vi "ToDatagram.vi"(8 "error in (no error)":errorcluster, 10 "messageID":u16, 11 "PublishCompleteMqttMsg in":refnum<class "PublishCompleteMqttMsg.lvclass">) -> (0 "error out":errorcluster, 2 "Datagram":u8[](array[numeric]), 3 "PublishCompleteMqttMsg out":refnum<class "PublishCompleteMqttMsg.lvclass">)   [LabVIEW 2020, in "PublishCompleteMqttMsg.lvclass"]
uses:
  PublishCompleteMqttMsg.lvclass
  mqttTypedef/mqttMessageType.ctl
  mqttTypedef/mqttQOSlevel.ctl
  PublishCompleteMqttMsg.lvclass/PublishCompleteMqttMsg.ctl
  BaseMqttMsg.lvclass
  mqtt.lvclass
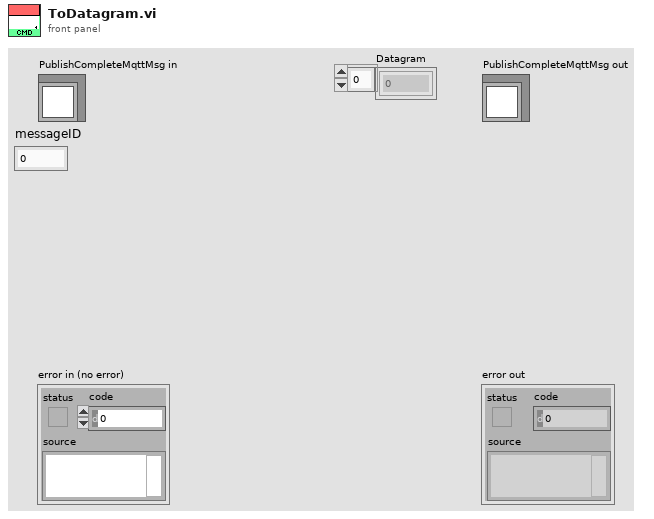
[diagram p1: front panel]
types:
  T1 = typedef "mqtt.lvclass/mqttQOSlevel.ctl" = enum8{"At most once", "At least once", "Exactly once", "Reserved"}
  T2 = typedef "mqtt.lvclass/mqttMessageType.ctl" = enum32{"Reserved", "CONNECT", "CONNACK", "PUBLISH", "PUBACK", "PUBREC", "PUBREL", "PUBCOMP", "SUBSCRIBE", "SUBACK", "UNSUBSCRIBE", "UNSUBACK", "PINGREQ", "PINGRESP", "DISCONNECT", "Reserved2"}
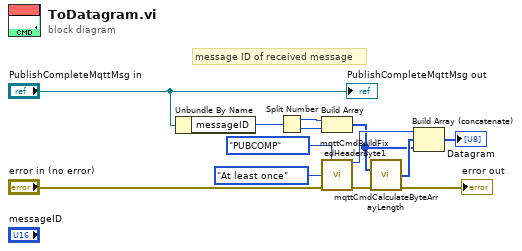
[diagram p0: block diagram]
diagram:
  # "message ID of received message"
  n1 = Unbundle By Name("PublishCompleteMqttMsg in") -> ("messageID"=w1:u16)
  n2 = Split Number(x=w1) -> (hi(x)=w9:u8, lo(x)=w10:u8)
  n3 = Build Array(w9, w10) -> (w8:u8[])
  n4 = call "mqttCmdBuildFixedHeaderByte1.vi"("MessageType"=mqttMessageType."PUBCOMP", "QoS (At most once)"=mqttQOSlevel."At least once", "error in (no error)"="error in (no error)") -> ("byte1"=w12:u8, "error out"=w13:errorcluster)  [unwired: 11 in]
  n5 = call "mqttCmdCalculateByteArrayLength.vi"("byteArry in"=w8, "error in (no error)"=w13) -> ("length out"=w11:u8[], "error out"=→"error out":errorcluster)  [unwired: 12 in]
  n6 = Build Array (concatenate)(w12, w11, w8) -> (→"Datagram":u8[])
  "PublishCompleteMqttMsg out" <- "PublishCompleteMqttMsg in"
